vi "FGV_EstadoEquipos.vi"(7 "Action":enum16{"Read", "Write"}(ring), 8 "Error In (no error)":errorcluster, 11 "Estado_Equipos":T2={"NOMBRE_EQUIPO"="PM_W02", "EstadoEquipo"="DESCONECTADO"}) -> (0 "Error Out":errorcluster, 3 "Estado_Equipos":T2)   [LabVIEW 2018]
uses:
  Controls/FGV_estadoequipos_action.ctl
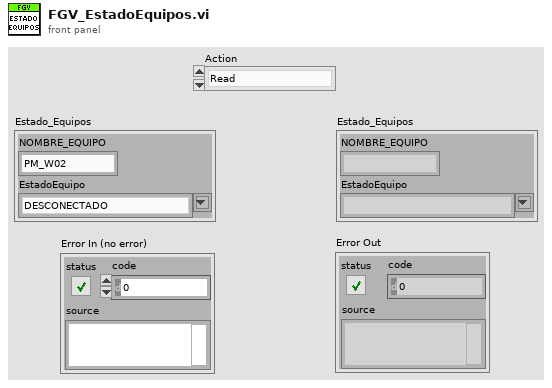
[diagram p1: front panel]
types:
  T1 = typedef "FGV_estadoequipos_action.ctl" = string
  T2 = cluster{"NOMBRE_EQUIPO":string, "EstadoEquipo":T1}
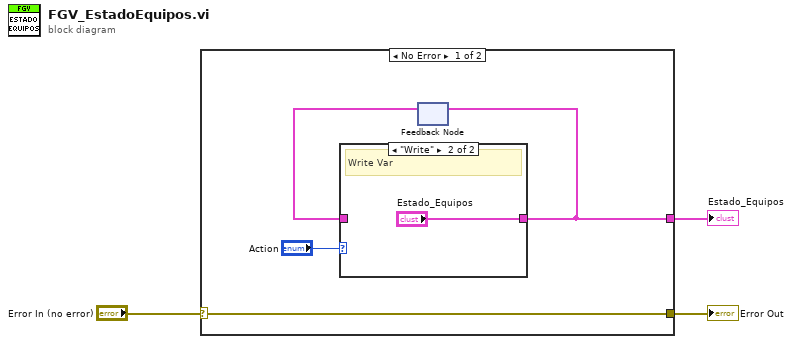
[diagram p0: block diagram]
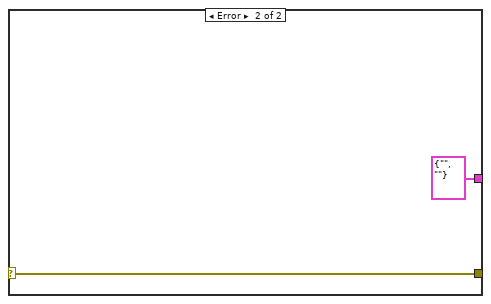
[diagram p3: hidden frame]
diagram:
  n1 = case shown="No Error" "Error In (no error)" {
    selector: "Error In (no error)" -> [w5 w11]
    tunnel: [w5 w11] -> w2
    tunnel: [w4 T2 {"NOMBRE_EQUIPO"="", "EstadoEquipo"=""} ("Estado_Equipos")] -> w1
    frame No Error {
      n2 = feedback #1() -> (w6:T2)  [unwired: 1 in]
      n3 = case shown="\"Write\"" "Action" {
        tunnel: [w8 "Estado_Equipos"] -> w4
        tunnel: w6 -> [w8 _]
        frame "Read", Default {
        }
        frame "Write" {
          # "Write Var"
        }
      }
      n4 = feedback-in #1(w4) -> ()
    }
    frame Error {
    }
  }
  "Error Out" <- w2
  "Estado_Equipos" <- w1
